vi "initGcode.vi"(6 "Che Do":bool=TRUE, 7 "gCode":T1, 8 "error in (no error)":errorcluster, 9 "PosSetG92":cluster{"X":dbl, "Y":dbl, "Z":dbl}, 10 "Gcode In":string, 11 "XuLyDataDisplay in":refnum<class "XuLyDataDisplay.lvclass">) -> (0 "error out":errorcluster, 2 "GcodeString Out":string, 3 "XuLyDataDisplay out":refnum<class "XuLyDataDisplay.lvclass">)   [LabVIEW 2014, in "LibraryGcode.lvlib" / "XuLyDataDisplay.lvclass"]
uses:
  XuLyDataDisplay.lvclass
  SelectGcode.ctl
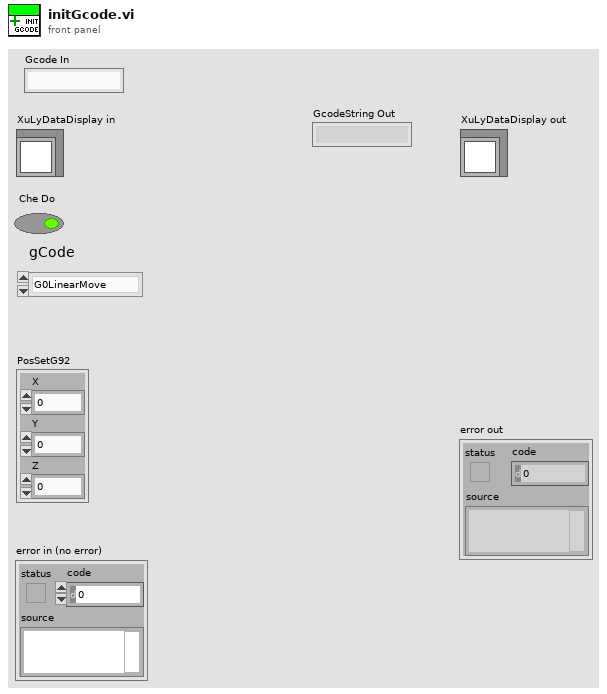
[diagram p1: front panel]
types:
  T1 = typedef "LibraryGcode.lvlib/XuLyDataDisplay.lvclass/SelectGcode.ctl" = enum16{"G0LinearMove", "G1XY", "G1LinearMove", "G2Arc", "G4Dwell", "G20InchUnit", "G21MilliUnit", "G28AutoHome", "G92SetPosition", "G90", "G91RelativePos", "JogX+", "JogX-", "JogY+", "JogY-", "JogZ+", "JogZ-", "sendGcodeString"}
  T2 = enum16{"Fan1", "Fan2", "Fan3", "PARA", "POS_DEGREE", "Solenoid", "Spindle", "TypeFirmware", "WaitPin", "MaxAcel", "MaxFeedrate", "MaxSize", "MaxStartAccel"}
  T3 = typedef "LibraryGcode.lvlib/TypeFirmwareControl.ctl" = enum16{"ScaraMarlin", "CncMarlin", "Mk4Due"}
  T4 = cluster{"PWM":dbl, "TypeFirmware":T3, "XYZ":cluster{"X":dbl, "Y":dbl, "Z":dbl}, "PARA":cluster{"STEP":i16, "FEEDRATE":dbl}, "DEGREES":cluster{"X":dbl, "Y":dbl}, "Solenoid":bool, "StartAccel":cluster{"P":dbl, "R":dbl, "T":dbl}}
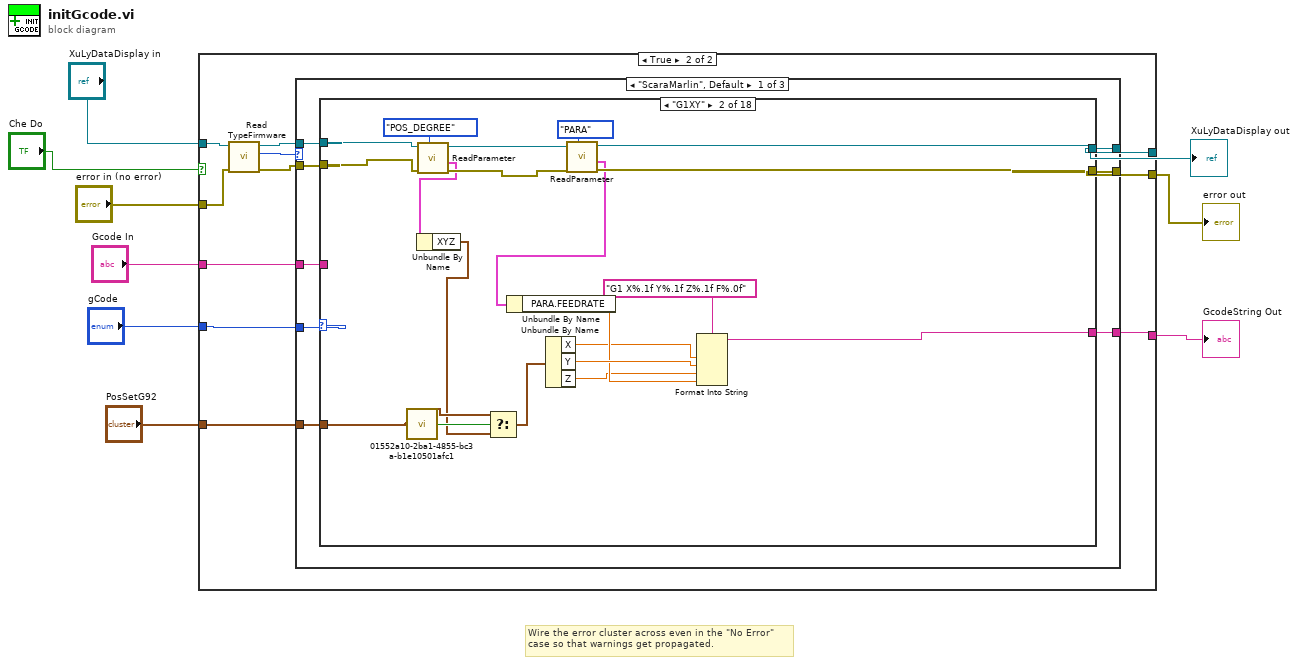
[diagram p0: block diagram]
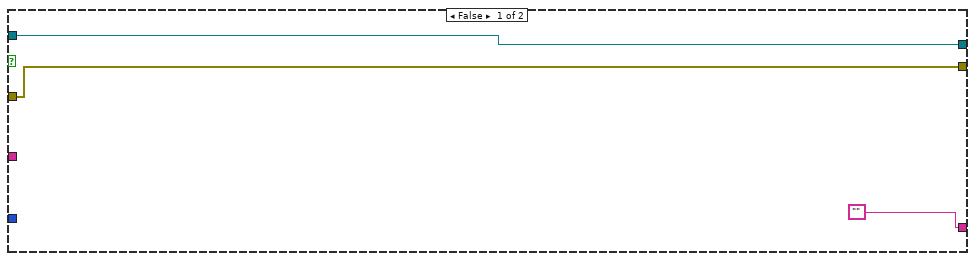
[diagram p2: hidden frame]
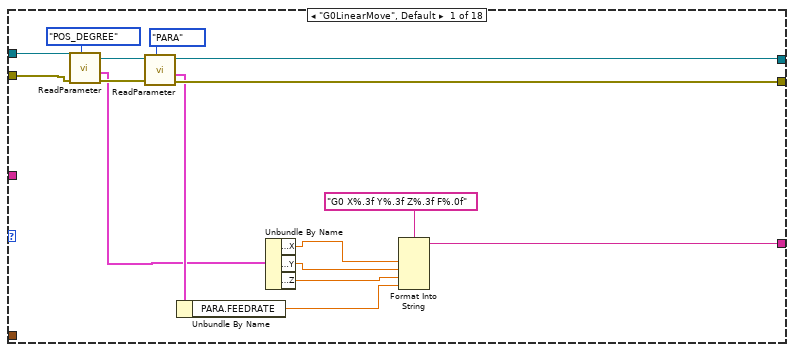
[diagram p3: hidden frame]
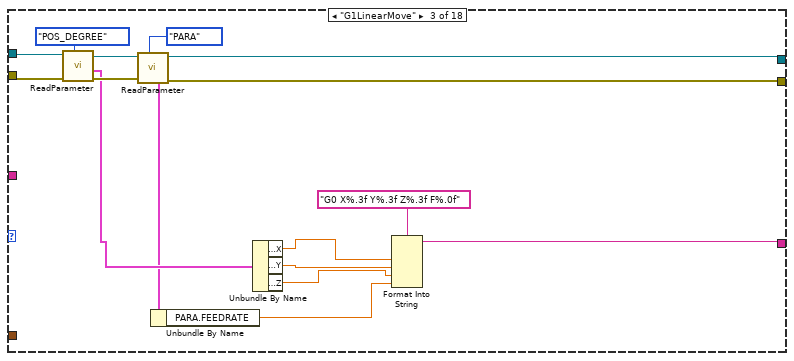
[diagram p4: hidden frame]
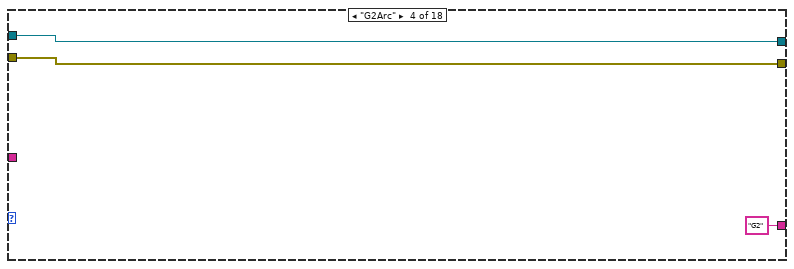
[diagram p5: hidden frame]
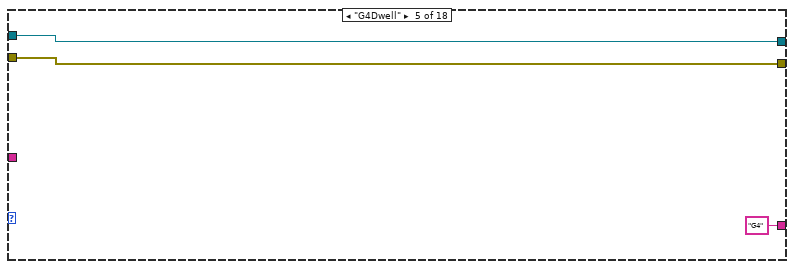
[diagram p6: hidden frame]
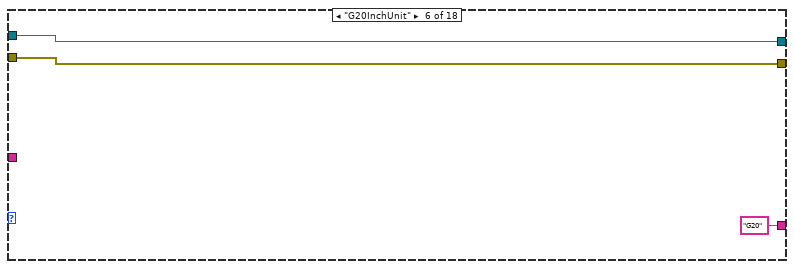
[diagram p7: hidden frame]
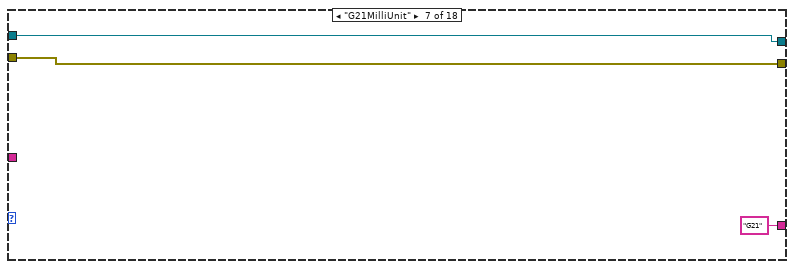
[diagram p8: hidden frame]
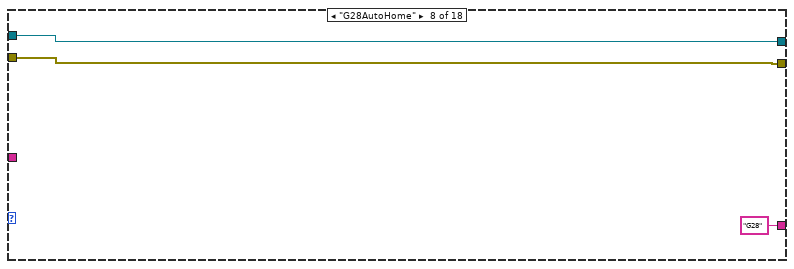
[diagram p9: hidden frame]
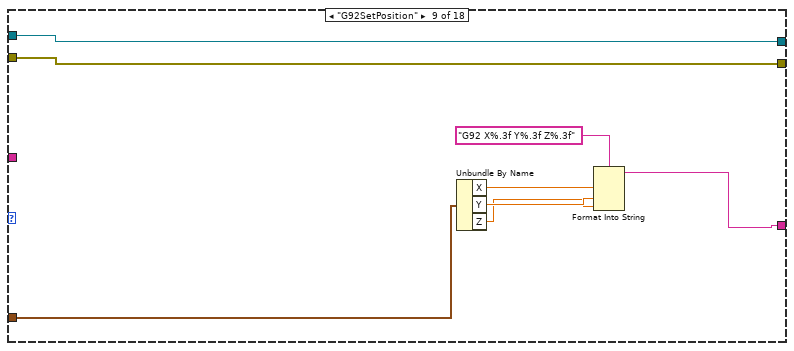
[diagram p10: hidden frame]
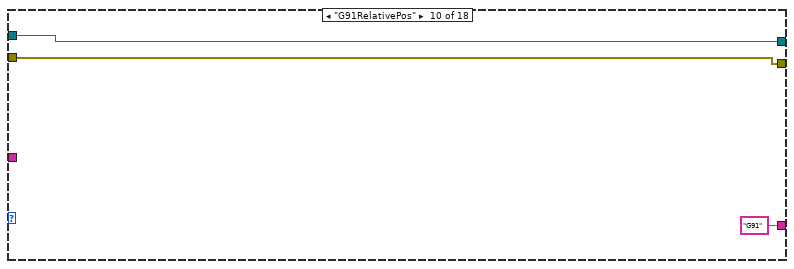
[diagram p11: hidden frame]
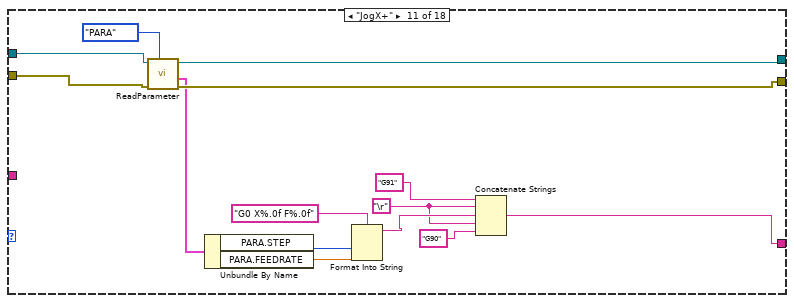
[diagram p12: hidden frame]
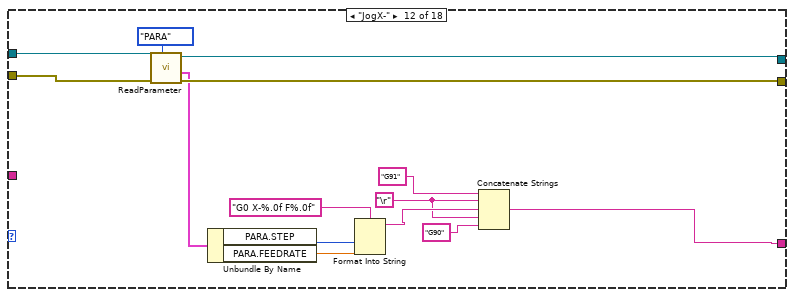
[diagram p13: hidden frame]
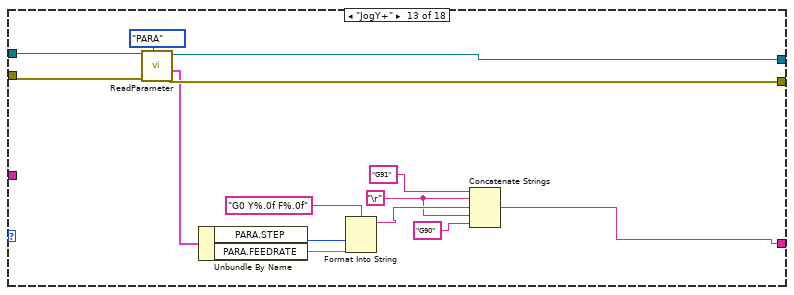
[diagram p14: hidden frame]
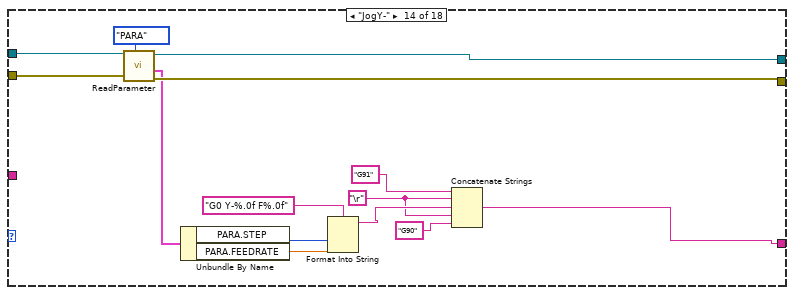
[diagram p15: hidden frame]
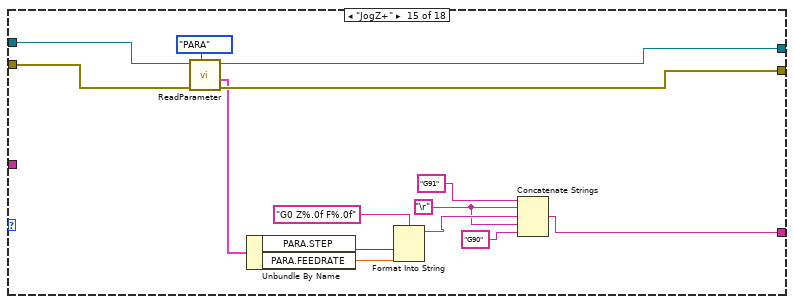
[diagram p16: hidden frame]
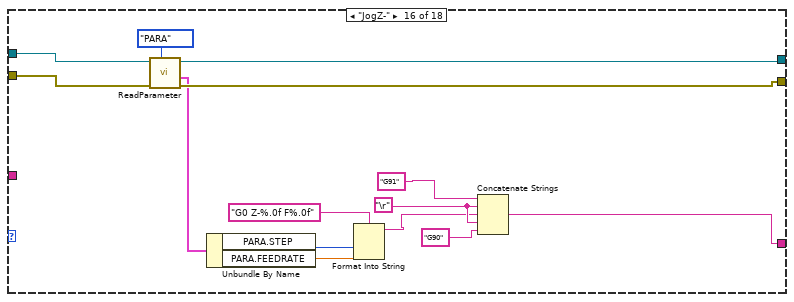
[diagram p17: hidden frame]
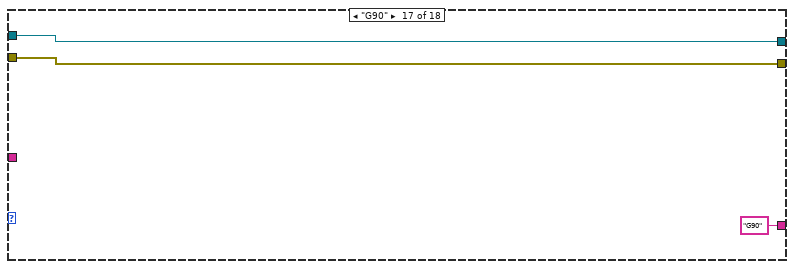
[diagram p18: hidden frame]
diagram:
  # "Wire the error cluster across even in the \"No Error\"\ncase so that warnings get propagated."
  n1 = case shown="True" "Che Do" {
    tunnel: [w11 w18] -> w9
    tunnel: [w12 w23] -> w8
    tunnel: "XuLyDataDisplay in" -> [w12 w21]
    tunnel: "gCode" -> [_ w17]
    tunnel: ["" w13] -> w5
    tunnel: "PosSetG92" -> [_ w16]
    tunnel: "error in (no error)" -> [w11 w15]
    tunnel: "Gcode In" -> [_ w14]
    frame False {
    }
    frame True {
      n2 = call-dynamic "Read TypeFirmware.vi"("error in (no error)"=w15, "ParameterConf in"=w21) -> ("error out"=w19:errorcluster, "TypeFirmware"=w20:T3, "ParameterConf out"=w22:refnum<class "XuLyDataDisplay.lvclass">)  [unwired: 7 in]
      n3 = case shown="\"ScaraMarlin\", Default" w20 {
        tunnel: [w28 w204 w210] -> w23
        tunnel: w22 -> [w27 w203 w210]
        tunnel: w19 -> [w29 w201 w209]
        tunnel: [w30 w202 w209] -> w18
        tunnel: w17 -> [w31 w200 _]
        tunnel: w16 -> [w26 _ _]
        tunnel: w14 -> [w24 _ _]
        tunnel: [w25 _ _] -> w13
        frame "ScaraMarlin", Default {
          n4 = case shown="\"G1XY\"" w31 {
            tunnel: [w38 w61 w74 w84 w87 w90 w93 w96 w99 w107 w113 w127 w142 w155 w170 w182 w194 w197] -> w30
            tunnel: w29 -> [w40 w58 w75 w84 w87 w90 w93 w96 w99 w107 w115 w129 w141 w157 w169 w187 w194 w197]
            tunnel: [w37 w62 w73 w85 w88 w91 w94 w97 w100 w108 w114 w128 w143 w156 w171 w183 w195 w198] -> w28
            tunnel: w27 -> [w43 w59 w76 w85 w88 w91 w94 w97 w100 w108 w116 w130 w144 w158 w172 w188 w195 w198]
            tunnel: [w36 w65 w72 "G2" "G4" "G20" "G21" "G28" w102 "G91" w112 w126 w140 w154 w168 w184 "G90" w199] -> w25
            tunnel: w26 -> [_ w63 _ _ _ _ _ _ w101 _ _ _ _ _ _ _ _ _]
            tunnel: w24 -> [_ _ _ _ _ _ _ _ _ _ _ _ _ _ _ _ _ w199]
            frame "G0LinearMove", Default {
              n5 = call-dynamic "ReadParameter.vi"("ParameterConf in"=w43, "error in (no error)"=w40, "Parameter"=T2."POS_DEGREE") -> ("ParameterConf out"=w42:refnum<class "XuLyDataDisplay.lvclass">, "DataOutClust"=w32:T4, "error out"=w39:errorcluster)  [unwired: 4 in, 1 out]
              n6 = call-dynamic "ReadParameter.vi"("ParameterConf in"=w42, "error in (no error)"=w39, "Parameter"=T2."PARA") -> ("ParameterConf out"=w37:refnum<class "XuLyDataDisplay.lvclass">, "DataOutClust"=w33:T4, "error out"=w38:errorcluster)  [unwired: 4 in, 1 out]
              n7 = Unbundle By Name(w33) -> ("PARA.FEEDRATE"=w41:dbl)
              n8 = Unbundle By Name(w32) -> ("XYZ.X"=w46:dbl, "XYZ.Y"=w45:dbl, "XYZ.Z"=w44:dbl)
              n9 = Format Into String(format string="G0 X%.3f Y%.3f Z%.3f F%.0f", w46, w45, w44, w41) -> (resulting string=w36:string)  [unwired: 2 in, 1 out]
            }
            frame "G1XY" {
              n10 = call "01552a10-2ba1-4855-bc3a-b1e10501afc1.vi"("value"=w63) -> ("changed or first call?"=w64:bool)
              n11 = call-dynamic "ReadParameter.vi"("ParameterConf in"=w59, "error in (no error)"=w58, "Parameter"=T2."POS_DEGREE") -> ("ParameterConf out"=w55:refnum<class "XuLyDataDisplay.lvclass">, "DataOutClust"=w53:T4, "error out"=w54:errorcluster)  [unwired: 4 in, 1 out]
              n12 = Unbundle By Name(w53) -> ("XYZ"=w52:cluster{"X":dbl, "Y":dbl, "Z":dbl})
              n13 = Select(t=w63, s=w64, f=w52) -> (s? t:f=w56:cluster{"X":dbl, "Y":dbl, "Z":dbl})
              n14 = Unbundle By Name(w56) -> ("X"=w48:dbl, "Y"=w66:dbl, "Z"=w49:dbl)
              n15 = call-dynamic "ReadParameter.vi"("ParameterConf in"=w55, "error in (no error)"=w54, "Parameter"=T2."PARA") -> ("ParameterConf out"=w62:refnum<class "XuLyDataDisplay.lvclass">, "DataOutClust"=w51:T4, "error out"=w61:errorcluster)  [unwired: 4 in, 1 out]
              n16 = Unbundle By Name(w51) -> ("PARA.FEEDRATE"=w50:dbl)
              n17 = Format Into String(format string="G1 X%.1f Y%.1f Z%.1f F%.0f", w48, w66, w49, w50) -> (resulting string=w65:string)  [unwired: 2 in, 1 out]
            }
            frame "G1LinearMove" {
              n18 = call-dynamic "ReadParameter.vi"("ParameterConf in"=w76, "error in (no error)"=w75, "Parameter"=T2."POS_DEGREE") -> ("ParameterConf out"=w79:refnum<class "XuLyDataDisplay.lvclass">, "DataOutClust"=w70:T4, "error out"=w77:errorcluster)  [unwired: 4 in, 1 out]
              n19 = call-dynamic "ReadParameter.vi"("ParameterConf in"=w79, "error in (no error)"=w77, "Parameter"=T2."PARA") -> ("ParameterConf out"=w73:refnum<class "XuLyDataDisplay.lvclass">, "DataOutClust"=w68:T4, "error out"=w74:errorcluster)  [unwired: 4 in, 1 out]
              n20 = Unbundle By Name(w68) -> ("PARA.FEEDRATE"=w78:dbl)
              n21 = Unbundle By Name(w70) -> ("XYZ.X"=w82:dbl, "XYZ.Y"=w81:dbl, "XYZ.Z"=w80:dbl)
              n22 = Format Into String(format string="G0 X%.3f Y%.3f Z%.3f F%.0f", w82, w81, w80, w78) -> (resulting string=w72:string)  [unwired: 2 in, 1 out]
            }
            frame "G2Arc" {
            }
            frame "G4Dwell" {
            }
            frame "G20InchUnit" {
            }
            frame "G21MilliUnit" {
            }
            frame "G28AutoHome" {
            }
            frame "G92SetPosition" {
              n23 = Unbundle By Name(w101) -> ("X"=w105:dbl, "Y"=w104:dbl, "Z"=w103:dbl)
              n24 = Format Into String(format string="G92 X%.3f Y%.3f Z%.3f", w105, w104, w103) -> (resulting string=w102:string)  [unwired: 2 in, 1 out]
            }
            frame "G91RelativePos" {
            }
            frame "JogX+" {
              w119 = "\r"
              n25 = call-dynamic "ReadParameter.vi"("ParameterConf in"=w116, "error in (no error)"=w115, "Parameter"=T2."PARA") -> ("ParameterConf out"=w114:refnum<class "XuLyDataDisplay.lvclass">, "DataOutClust"=w110:T4, "error out"=w113:errorcluster)  [unwired: 4 in, 1 out]
              n26 = Unbundle By Name(w110) -> ("PARA.STEP"=w122:i16, "PARA.FEEDRATE"=w121:dbl)
              n27 = Format Into String(format string="G0 X%.0f F%.0f", w122, w121) -> (resulting string=w123:string)  [unwired: 2 in, 1 out]
              n28 = Concatenate Strings("G91" ("string"), w119, w123, w119, "G90" ("string")) -> (w112:string)
            }
            frame "JogX-" {
              w133 = "\r"
              n29 = call-dynamic "ReadParameter.vi"("ParameterConf in"=w130, "error in (no error)"=w129, "Parameter"=T2."PARA") -> ("ParameterConf out"=w128:refnum<class "XuLyDataDisplay.lvclass">, "DataOutClust"=w125:T4, "error out"=w127:errorcluster)  [unwired: 4 in, 1 out]
              n30 = Unbundle By Name(w125) -> ("PARA.STEP"=w136:i16, "PARA.FEEDRATE"=w135:dbl)
              n31 = Format Into String(format string="G0 X-%.0f F%.0f", w136, w135) -> (resulting string=w137:string)  [unwired: 2 in, 1 out]
              n32 = Concatenate Strings("G91" ("string"), w133, w137, w133, "G90" ("string")) -> (w126:string)
            }
            frame "JogY+" {
              w147 = "\r"
              n33 = call-dynamic "ReadParameter.vi"("ParameterConf in"=w144, "error in (no error)"=w141, "Parameter"=T2."PARA") -> ("ParameterConf out"=w143:refnum<class "XuLyDataDisplay.lvclass">, "DataOutClust"=w139:T4, "error out"=w142:errorcluster)  [unwired: 4 in, 1 out]
              n34 = Unbundle By Name(w139) -> ("PARA.STEP"=w150:i16, "PARA.FEEDRATE"=w149:dbl)
              n35 = Format Into String(format string="G0 Y%.0f F%.0f", w150, w149) -> (resulting string=w151:string)  [unwired: 2 in, 1 out]
              n36 = Concatenate Strings("G91" ("string"), w147, w151, w147, "G90" ("string")) -> (w140:string)
            }
            frame "JogY-" {
              w161 = "\r"
              n37 = call-dynamic "ReadParameter.vi"("ParameterConf in"=w158, "error in (no error)"=w157, "Parameter"=T2."PARA") -> ("ParameterConf out"=w156:refnum<class "XuLyDataDisplay.lvclass">, "DataOutClust"=w153:T4, "error out"=w155:errorcluster)  [unwired: 4 in, 1 out]
              n38 = Unbundle By Name(w153) -> ("PARA.STEP"=w164:i16, "PARA.FEEDRATE"=w165:dbl)
              n39 = Format Into String(format string="G0 Y-%.0f F%.0f", w164, w165) -> (resulting string=w163:string)  [unwired: 2 in, 1 out]
              n40 = Concatenate Strings("G91" ("string"), w161, w163, w161, "G90" ("string")) -> (w154:string)
            }
            frame "JogZ+" {
              w175 = "\r"
              n41 = call-dynamic "ReadParameter.vi"("ParameterConf in"=w172, "error in (no error)"=w169, "Parameter"=T2."PARA") -> ("ParameterConf out"=w171:refnum<class "XuLyDataDisplay.lvclass">, "DataOutClust"=w167:T4, "error out"=w170:errorcluster)  [unwired: 4 in, 1 out]
              n42 = Unbundle By Name(w167) -> ("PARA.STEP"=w178:i16, "PARA.FEEDRATE"=w179:dbl)
              n43 = Format Into String(format string="G0 Z%.0f F%.0f", w178, w179) -> (resulting string=w177:string)  [unwired: 2 in, 1 out]
              n44 = Concatenate Strings("G91" ("string"), w175, w177, w175, "G90" ("string")) -> (w168:string)
            }
            frame "JogZ-" {
              w193 = "\r"
              n45 = call-dynamic "ReadParameter.vi"("ParameterConf in"=w188, "error in (no error)"=w187, "Parameter"=T2."PARA") -> ("ParameterConf out"=w183:refnum<class "XuLyDataDisplay.lvclass">, "DataOutClust"=w181:T4, "error out"=w182:errorcluster)  [unwired: 4 in, 1 out]
              n46 = Unbundle By Name(w181) -> ("PARA.STEP"=w186:i16, "PARA.FEEDRATE"=w185:dbl)
              n47 = Format Into String(format string="G0 Z-%.0f F%.0f", w186, w185) -> (resulting string=w189:string)  [unwired: 2 in, 1 out]
              n48 = Concatenate Strings("G91" ("string"), w193, w189, w193, "G90" ("string")) -> (w184:string)
            }
            frame "G90" {
            }
            frame "sendGcodeString" {
            }
          }
        }
        frame "CncMarlin" {
          n49 = case shown="\"G1XY\"" w200 {
            tunnel: [w206 w208] -> w204
            tunnel: w203 -> [w206 w208]
            tunnel: [w205 w207] -> w202
            tunnel: w201 -> [w205 w207]
            frame "G0LinearMove", Default {
            }
            frame "G1XY" {
            }
          }
        }
        frame "Mk4Due" {
        }
      }
    }
  }
  "error out" <- w9
  "XuLyDataDisplay out" <- w8
  "GcodeString Out" <- w5
